vi "Geometry Definition - Orient3d.vi"(4 "Feature Name":string, 6 "Part Type":string, 7 "Get/Set":enum16{"Get", "Set"}(ring), 8 "error in (no error)":errorcluster, 9 "Geometry Definition in":refnum<class "Orient3d.lvclass">, 11 "FlexWorktable in":refnum<class "FlexWorktable.lvclass">) -> (0 "error out":errorcluster, 1 "Geometry Definition out":refnum<class "Orient3d.lvclass">, 3 "FlexWorktable out":refnum<class "FlexWorktable.lvclass">)   [LabVIEW 2024, in "FlexWorktable.lvclass"]
uses:
  FlexWorktable.lvclass
  Orient3d Class/Orient3d.lvclass
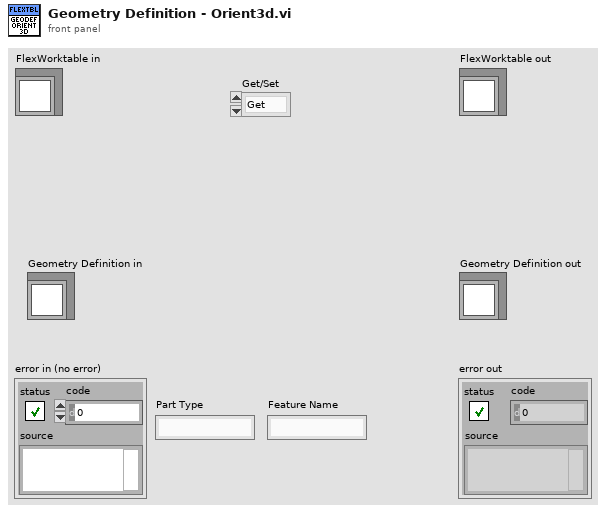
[diagram p1: front panel]
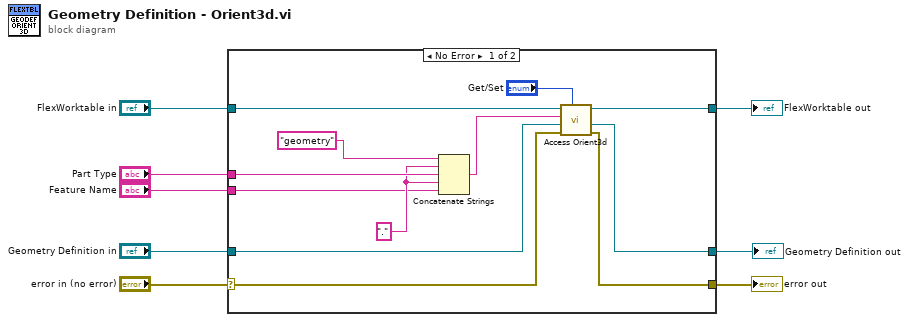
[diagram p0: block diagram]
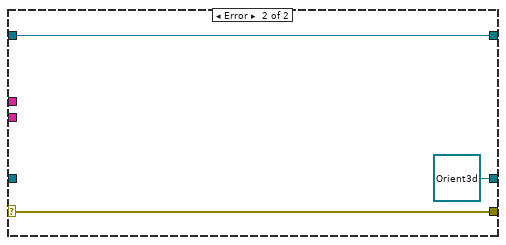
[diagram p2: hidden frame]
diagram:
  n1 = case shown="No Error" "error in (no error)" {
    selector: "error in (no error)" -> [w16 w23]
    tunnel: [w15 w23] -> w7
    tunnel: [w19 w22] -> w5
    tunnel: "FlexWorktable in" -> [w20 w22]
    tunnel: "Part Type" -> [w12 _]
    tunnel: "Feature Name" -> [w10 _]
    tunnel: "Geometry Definition in" -> [w17 _]
    tunnel: [w14 refnum<class "Orient3d.lvclass"> refnum ("Value out")] -> w2
    frame No Error {
      w11 = "."
      n2 = Concatenate Strings("geometry", w11, w12, w11, w10) -> (w9:string)
      n3 = call-dynamic "Access Orient3d.vi"("Get/Set"="Get/Set", "error in (no error)"=w16, "Value in"=w17, "Key"=w9, "FlexWorktable in"=w20) -> ("error out"=w15:errorcluster, "Value out"=w14:refnum<class "Orient3d.lvclass">, "FlexWorktable out"=w19:refnum<class "FlexWorktable.lvclass">)  [unwired: 4 in]
    }
    frame Error {
    }
  }
  "error out" <- w7
  "FlexWorktable out" <- w5
  "Geometry Definition out" <- w2
